vi "main.vi"() -> ()   [LabVIEW 2016]
uses:
  System Status.ctl
  Position Control.ctl
  Position Coordinate.ctl
  Manual Operation Control.ctl
  <vilib>/MakerHub/Xbox-One-Controller/Public/Open First Controller.vi
  <vilib>/MakerHub/Xbox-One-Controller/LMH-Xbox-One-Controller.lvlib
panel:
  in  "Exit Controller":bool
  in  "Use Controller":bool
  out "Numeric 2":dbl
  in  "MotionIni File In":path=path "C:/Program Files (x86)/National Instruments/LabVIEW 2016/user.lib/iselmotion/CNCAPI/CtrlDll/Dummy/MctlDummy.INI"
  in  "MotionLibrary Path":path=path "C:/Program Files (x86)/National Instruments/LabVIEW 2016/user.lib/iselmotion/CNCAPI/CtrlDll/Dummy/mctlDummy.dll"
  in  "Auto Run Control":T1[](array[typedef])
  in  "Auto Run":bool
  in  "Abs Position":T2={"Pos X"=0.0, "Position Name"="Abs Move", "Pos Y"=0.0, "Pos Z"=0.0, "Pos A"=0.0, "OK Button"=FALSE, "Normal Move"=FALSE, "Fast Move"=FALSE} {"Pos A" format="%.2f"; "Pos Z" format="%.2f"; "Pos Y" format="%.2f"; "Pos X" format="%.2f"}
  in  "Rel Position":T2={"Pos X"=0.0, "Position Name"="Rel Move", "Pos Y"=0.0, "Pos Z"=0.0, "Pos A"=0.0, "OK Button"=FALSE, "Normal Move"=FALSE, "Fast Move"=FALSE} {"Pos A" format="%.2f"; "Pos Z" format="%.2f"; "Pos Y" format="%.2f"; "Pos X" format="%.2f"}
  in  "Manual Operation Control":T3={"Pos X"={"Plus"=FALSE, "Minus"=FALSE}, "Pos Y"={"Plus"=FALSE, "Minus"=FALSE}, "Pos Z"={"Plus"=FALSE, "Minus"=FALSE}, "Pos A"={"Plus"=FALSE, "Minus"=FALSE}, "Linear"={"Speed"=1.0, "Step Length"=0.01}, "Rotative"={"Speed"=1.0, "Step Length"=0.01}, "Speed Override (%)"=100.0, "Axis-A Movement"=FALSE} {"Speed Override (%)" min=0.0 max=150.0 step=1.0 scale=0.0..150.0; "Rotative"."Step Length" min=0.01 max=100.0 step=0.01; "Rotative"."Speed" min=0.0 max=500.0 step=1.0 scale=0.0..500.0 scale format="%#.0f"; "Linear"."Step Length" min=0.01 max=500.0 step=0.01; "Linear"."Speed" min=0.0 max=500.0 step=1.0 scale=0.0..500.0 scale format="%#.0f"}
  out "Status":bool
  in  "Test Mode":bool
  in  "Leave HWLS":bool
  in  "Reference":bool
  in  "Reset Motion":bool
  in  "Stop Motion":bool
  in  "Settings":bool
  in  "Exit":bool
  in  "Initialize":bool
  out "System Status":T4 {"Axis A"."Position" format="%.2f"; "Axis Z"."Position" format="%.2f"; "Axis Y"."Position" format="%.2f"; "Rotativ Speed" format="%#_6f"; "Linear Speed" format="%#.2f"; "Axis X"."Position" format="%.2f"}
  out "Error Information":string
  out "Motor hModule":i32
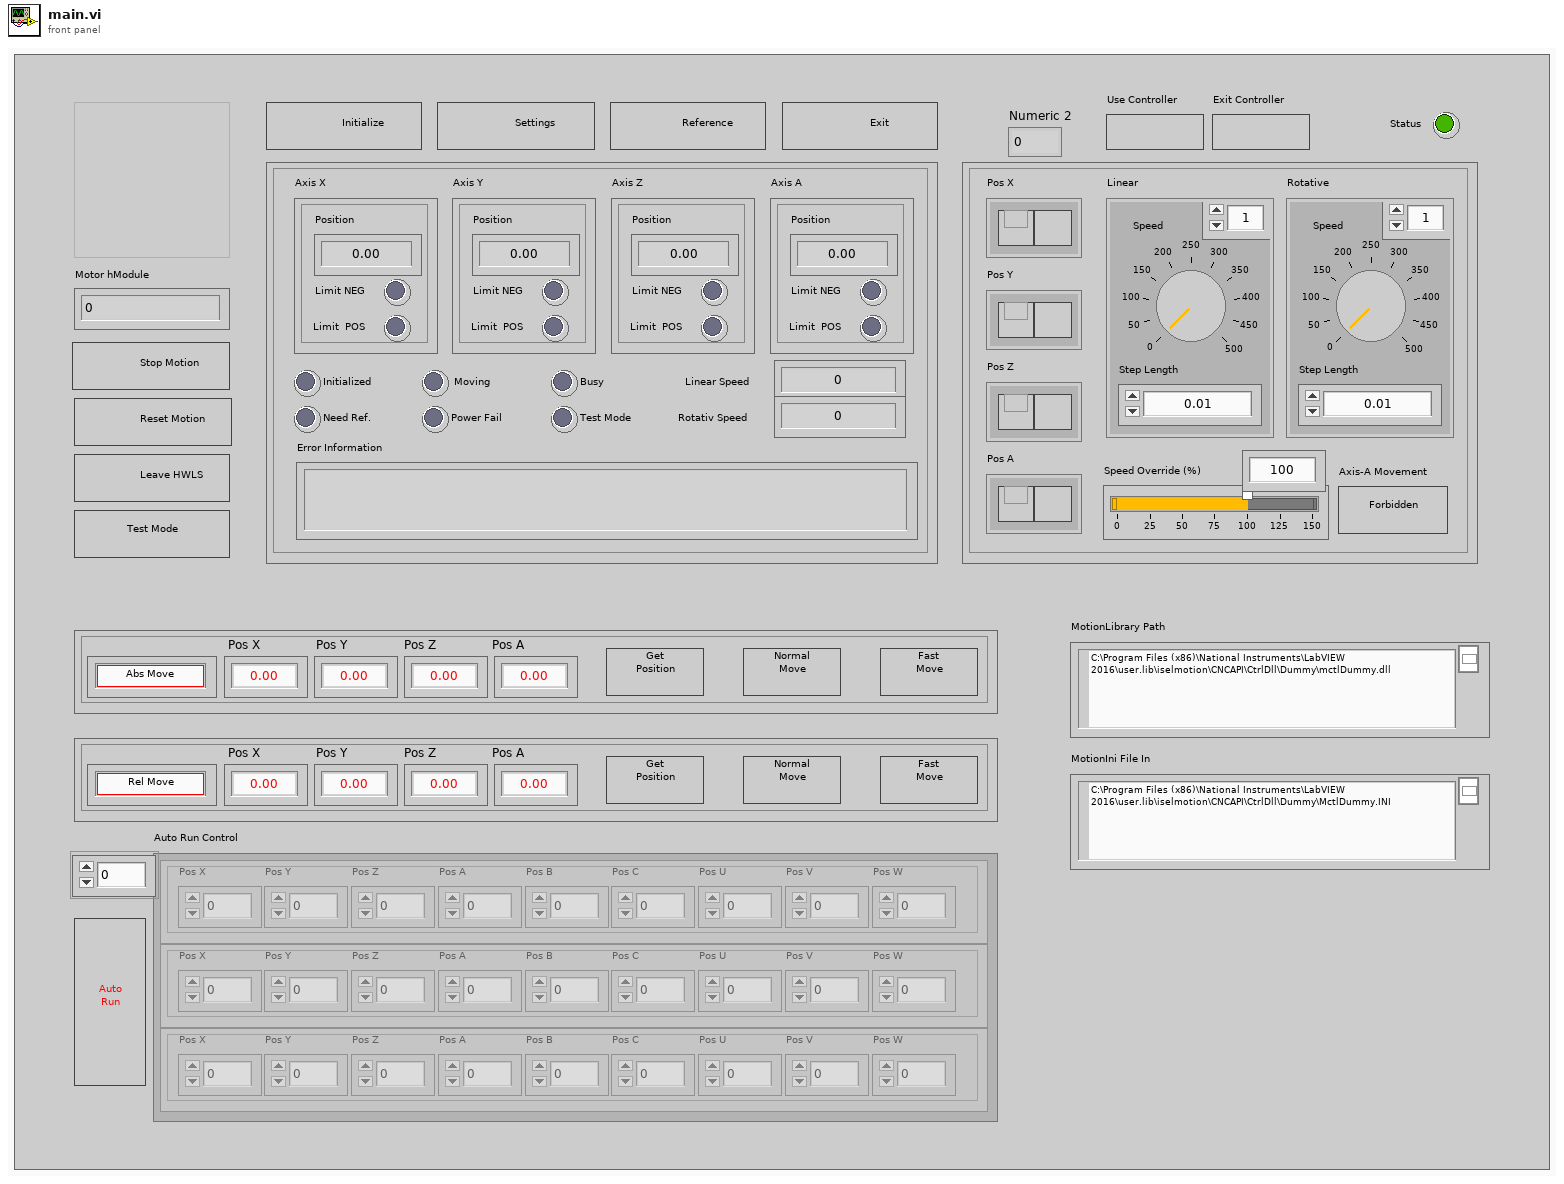
[diagram p1: front panel]
types:
  T1 = typedef "Position Coordinate.ctl" = cluster{"Pos X":dbl, "Pos Y":dbl, "Pos Z":dbl, "Pos A":dbl, "Pos B":dbl, "Pos C":dbl, "Pos U":dbl, "Pos V":dbl, "Pos W":dbl}
  T2 = typedef "Position Control.ctl" = cluster{"Pos X":dbl, "Position Name":string, "Pos Y":dbl, "Pos Z":dbl, "Pos A":dbl, "OK Button":bool, "Normal Move":bool, "Fast Move":bool}
  T3 = typedef "Manual Operation Control.ctl" = cluster{"Pos X":cluster{"Plus":bool, "Minus":bool}, "Pos Y":cluster{"Plus":bool, "Minus":bool}, "Pos Z":cluster{"Plus":bool, "Minus":bool}, "Pos A":cluster{"Plus":bool, "Minus":bool}, "Linear":cluster{"Speed":dbl, "Step Length":dbl}, "Rotative":cluster{"Speed":dbl, "Step Length":dbl}, "Speed Override (%)":dbl, "Axis-A Movement":bool}
  T4 = typedef "System Status.ctl" = cluster{"Axis X":cluster{"Position":dbl, "Limit NEG":bool, "Limit  POS":bool}, "Axis Y":cluster{"Position":dbl, "Limit NEG":bool, "Limit  POS":bool}, "Axis Z":cluster{"Position":dbl, "Limit NEG":bool, "Limit  POS":bool}, "Axis A":cluster{"Position":dbl, "Limit NEG":bool, "Limit  POS":bool}, "Initialized":bool, " Moving":bool, "Busy":bool, "Need Ref.":bool, "Power Fail":bool, "Test Mode":bool, "Linear Speed":dbl, "Rotativ Speed":dbl, "Error Information":string}
  T5 = enum16{"open", "replace", "create", "open or create", "replace or create", "replace or create with confirmation"}
  T6 = enum8{"Enabled", "Disabled", "Disabled and Grayed Out"}
  T7 = cluster{"PosX":i32, "PosY":i32, "PosZ":i32, "PosA":i32, "PosB":i32, "PosC":i32, "PosU":i32, "PosV":i32, "PosW":i32}
  T8 = cluster{"MotionLibrary Path":path, "MotionIni File In":path}
  T9 = typedef "LMH-Xbox-One-Controller.lvlib/Xbox One Controller Ref.ctl" = cluster{"Controller Ref":refnum<k1>, "Event Refnum":refnum<event-registration>, "Worker Ref":refnum<vi>}
  T10 = cluster{"Common":cluster{"INMOTION":bool, "INSTOPMODE":bool, "INTEACHMODE":bool, "INTESTMODE":bool, "CURRENTOFF":bool, "INPATHMOTION":bool, "ISMOVING":bool, "PATHSTARTED":bool, "NEEDREFERENCERUN":bool, "BREAKERROR":bool, "HWLSACTIVE":bool, "SWLSACTIVE":bool, "HWLSDURINGMOTION":bool, "AFTERRUNERROR":bool, "LOADPATHDATAERROR":bool, "KEYSWITCHERROR":bool, "KEYSWDURINGMOTION":bool, "POWER_FAIL":bool, "SC_FAIL":bool, "HARDWARE_FAIL":bool, "COMMUNICATION_FAIL":bool}, "HWLSNeg":cluster{"HWLS_X_NEG":bool, "HWLS_Y_NEG":bool, "HWLS_Z_NEG":bool, "HWLS_A_NEG":bool, "HWLS_B_NEG":bool, "HWLS_C_NEG":bool, "HWLS_U_NEG":bool, "HWLS_V_NEG":bool, "HWLS_W_NEG":bool}, "HWLSPos":cluster{"HWLS_X_POS":bool, "HWLS_Y_POS":bool, "HWLS_Z_POS":bool, "HWLS_A_POS":bool, "HWLS_B_POS":bool, "HWLS_C_POS":bool, "HWLS_U_POS":bool, "HWLS_V_POS":bool, "HWLS_W_POS":bool}, "SWLSNeg":cluster{"SWLS_X_NEG":bool, "SWLS_Y_NEG":bool, "SWLS_Z_NEG":bool, "SWLS_A_NEG":bool, "SWLS_B_NEG":bool, "SWLS_C_NEG":bool, "SWLS_U_NEG":bool, "SWLS_V_NEG":bool, "SWLS_W_NEG":bool}, "SWLSPos":cluster{"SWLS_X_POS":bool, "SWLS_Y_POS":bool, "SWLS_Z_POS":bool, "SWLS_A_POS":bool, "SWLS_B_POS":bool, "SWLS_C_POS":bool, "SWLS_U_POS":bool, "SWLS_V_POS":bool, "SWLS_W_POS":bool}, "Extended":cluster{"ISBUSY":bool, "DISABLED":bool, "ISINITIALIZED":bool, "READY":bool, "DRILLCYCLEACTIVE":bool, "CTRLSPECERROR":bool}, "Additional flags":cluster{"InMotion":bool, "InStopMode":bool, "InTeachMode":bool, "InTestMode":bool, "CurrentOff":bool, "InPathMotion":bool, "IsMoving":bool, "NeedReferenceRun":bool, "BreakError":bool, "HWLSActive":bool, "SWLSActive":bool, "HWLSDuringMotion":bool, "AfterRunError":bool, "PowerFail":bool, "SCFail":bool, "IsBusy":bool, "Initialized":bool, "Disabled":bool, "HardwareFail":bool, "CommunicationFail":bool, "DrillCycleActive":bool, "CtrlSpecError":bool, "PathStarted":bool}}
  T11 = cluster{"PosX":dbl, "PosY":dbl, "PosZ":dbl, "PosA":dbl, "PosB":dbl, "PosC":dbl, "PosU":dbl, "PosV":dbl, "PosW":dbl}
  T12 = cluster{"PosX":dbl, "HWLS_X_NEG":bool, "HWLS_X_POS":bool}
  T13 = cluster{"PosY":dbl, "HWLS_Y_NEG":bool, "HWLS_Y_POS":bool}
  T14 = cluster{"PosZ":dbl, "HWLS_Z_NEG":bool, "HWLS_Z_POS":bool}
  T15 = cluster{dbl, "HWLS_A_NEG":bool, "HWLS_A_POS":bool}
  T16 = cluster{"LiNormVel":i32, "DrNormVel":i32, "LiFastVel":i32, "DrFastVel":i32, "LiTeachVel":i32, "DrTeachVel":i32, "LiActVel":i32, "DrActVel":i32}
  T17 = cluster{"LiNormVel":dbl, "DrNormVel":dbl, "LiFastVel":dbl, "DrFastVel":dbl, "LiTeachVel":dbl, "DrTeachVel":dbl, "LiActVel":dbl, "DrActVel":dbl}
  T18 = typedef "LMH-Xbox-One-Controller.lvlib/All Buttons Visual.ctl" = cluster{"A":T19, "B":T20, "X":T21, "Y":T22, "Left Bumper":T23, "Right Bumper":T24, "View Button":T25, "Menu Button":T26, "Left Stick":T27, "Right Stick":T27}
  T19 = typedef "LMH-Xbox-One-Controller.lvlib/A.ctl" = bool
  T20 = typedef "LMH-Xbox-One-Controller.lvlib/B.ctl" = bool
  T21 = typedef "LMH-Xbox-One-Controller.lvlib/X.ctl" = bool
  T22 = typedef "LMH-Xbox-One-Controller.lvlib/Y.ctl" = bool
  T23 = typedef "LMH-Xbox-One-Controller.lvlib/Left Bumper.ctl" = bool
  T24 = typedef "LMH-Xbox-One-Controller.lvlib/Right Bumper.ctl" = bool
  T25 = typedef "LMH-Xbox-One-Controller.lvlib/View.ctl" = bool
  T26 = typedef "LMH-Xbox-One-Controller.lvlib/Menu.ctl" = bool
  T27 = typedef "LMH-Xbox-One-Controller.lvlib/Thumbstick.ctl" = bool
  T28 = typedef "LMH-Xbox-One-Controller.lvlib/All Axis Data.ctl" = cluster{"Left Stick":cluster{"X Axis":i32, "Y Axis":i32}, "Right Stick":cluster{"X Axis":i32, "Y Axis":i32}, "Triggers":i32, "D-Pad":T29}
  T29 = typedef "LMH-Xbox-One-Controller.lvlib/DPad Enum.ctl" = enum16{"Idle", "Up", "Up / Right", "Right", "Down / Right", "Down", "Down / Left", "Left", "Up / Left"}
  T30 = cluster{"X Axis":i32, "Y Axis":i32, "Y Axis":i32, "Triggers":i32}
  T31 = cluster{"X Axis":bool, "Y Axis":bool, "Y Axis":bool, "Triggers":bool}
  T32 = cluster{"[0]":dbl, "[1]":dbl, "[2]":dbl, "[3]":dbl}
  T33 = cluster{"Ability":cluster{"LINEAR":bool, "CIRCLE":bool, "HELIX":bool, "SPLINE":bool, "BEZIER":bool, "PRECALC":bool, "ONLINE":bool}, "NumAxis":u32, "AxisConfig":cluster{"AxisConfig 0":cluster{"Type":cluster{"LINEAR":bool, "ROT":bool}, "In Use":bool, "ID":u32, "RangeMin":u32, "RangeMax":u32}, "AxisConfig 1":cluster{"Type":cluster{"LINEAR":bool, "ROT":bool}, "In Use":bool, "ID":u32, "RangeMin":u32, "RangeMax":u32}, "AxisConfig 2":cluster{"Type":cluster{"LINEAR":bool, "ROT":bool}, "In Use":bool, "ID":u32, "RangeMin":u32, "RangeMax":u32}, "AxisConfig 3":cluster{"Type":cluster{"LINEAR":bool, "ROT":bool}, "In Use":bool, "ID":u32, "RangeMin":u32, "RangeMax":u32}, "AxisConfig 4":cluster{"Type":cluster{"LINEAR":bool, "ROT":bool}, "In Use":bool, "ID":u32, "RangeMin":u32, "RangeMax":u32}, "AxisConfig 5":cluster{"Type":cluster{"LINEAR":bool, "ROT":bool}, "In Use":bool, "ID":u32, "RangeMin":u32, "RangeMax":u32}, "AxisConfig 6":cluster{"Type":cluster{"LINEAR":bool, "ROT":bool}, "In Use":bool, "ID":u32, "RangeMin":u32, "RangeMax":u32}, "AxisConfig 7":cluster{"Type":cluster{"LINEAR":bool, "ROT":bool}, "In Use":bool, "ID":u32, "RangeMin":u32, "RangeMax":u32}, "AxisConfig 8":cluster{"Type":cluster{"LINEAR":bool, "ROT":bool}, "In Use":bool, "ID":u32, "RangeMin":u32, "RangeMax":u32}}}
  T34 = cluster{"In Use":bool, "In Use":bool, "In Use":bool, "In Use":bool, "In Use":bool, "In Use":bool, "In Use":bool, "In Use":bool, "In Use":bool}
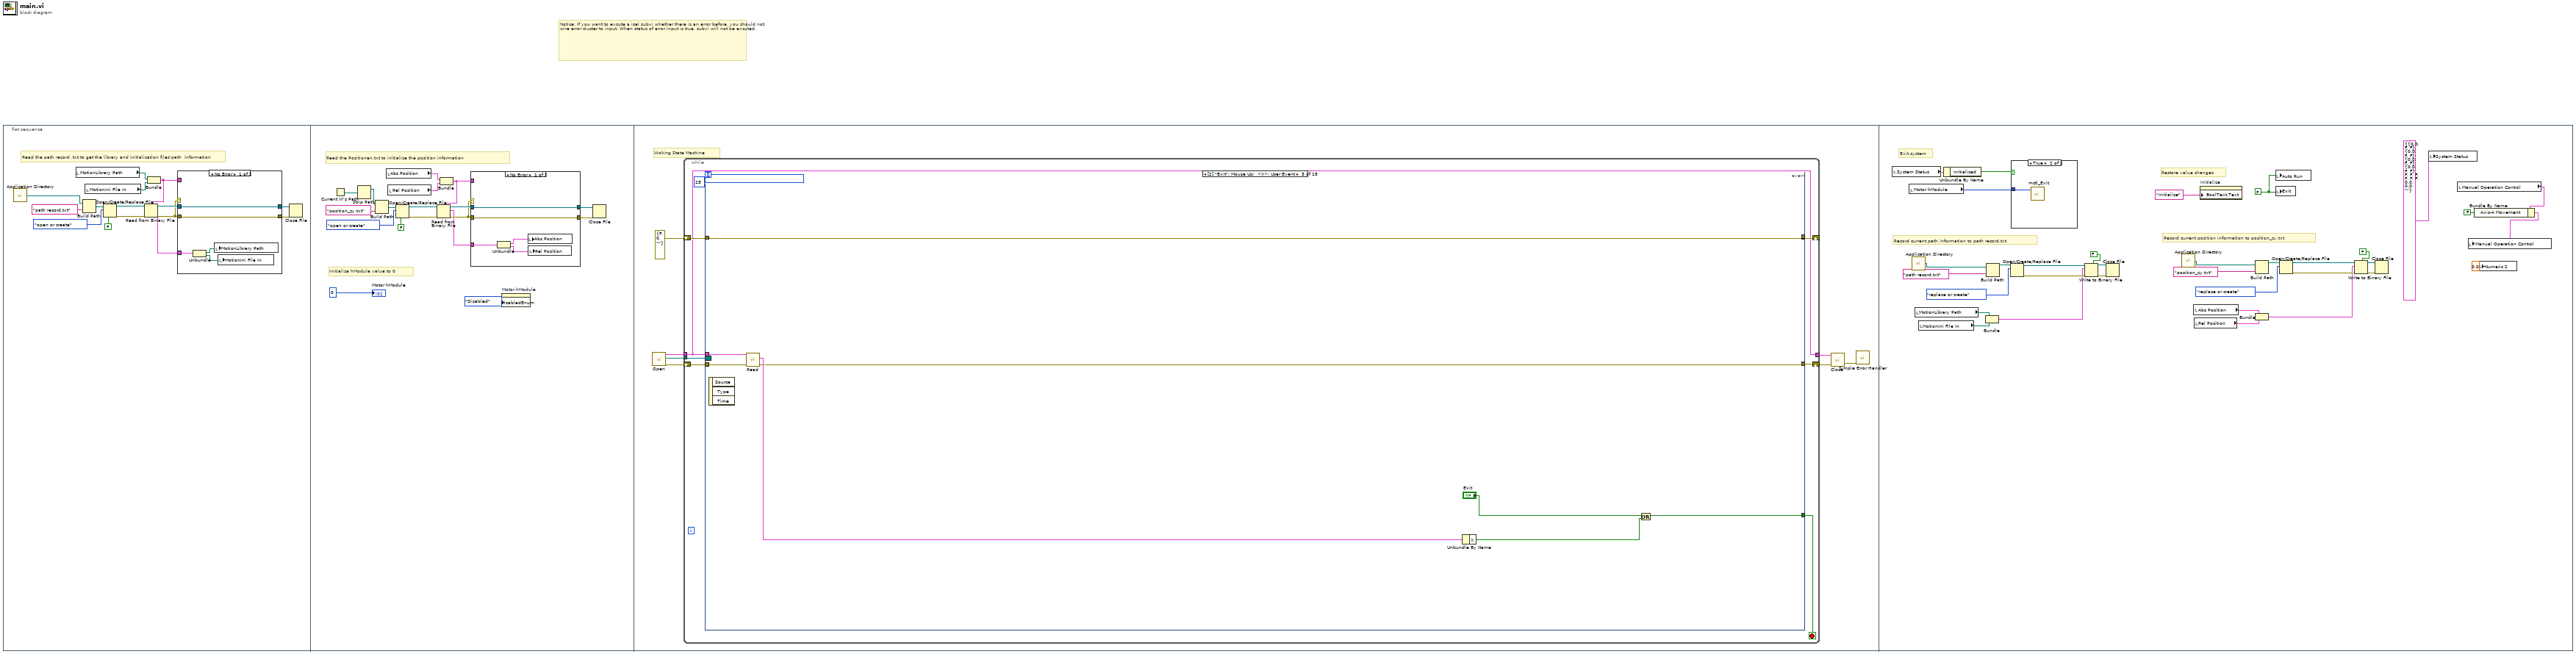
[diagram p0: block diagram]
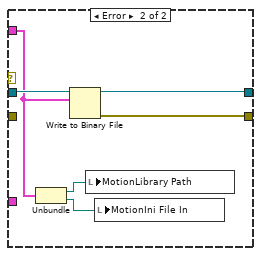
[diagram p2: hidden frame]
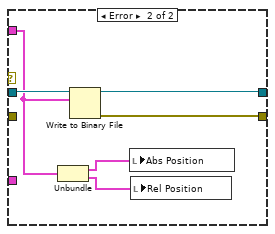
[diagram p3: hidden frame]
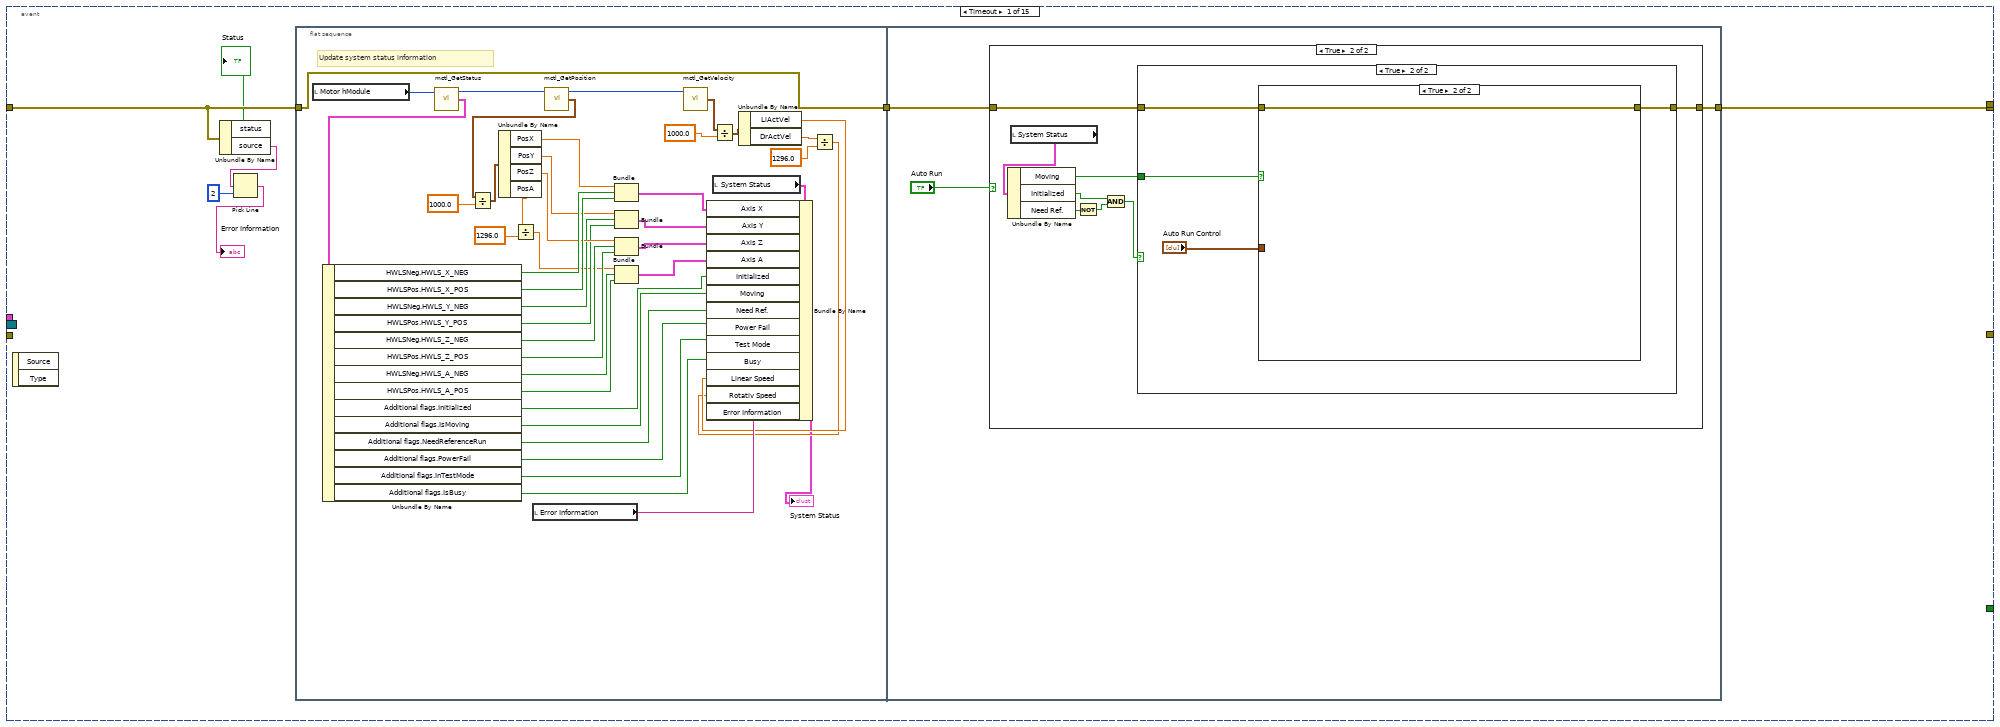
[diagram p4: hidden frame]
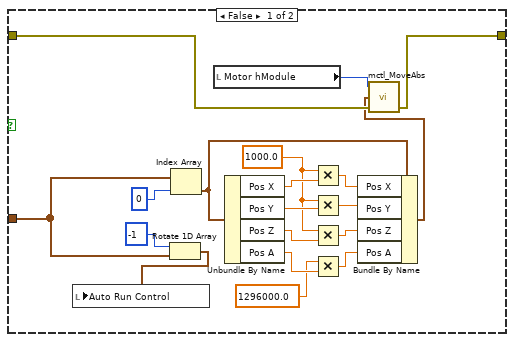
[diagram p7: hidden frame]
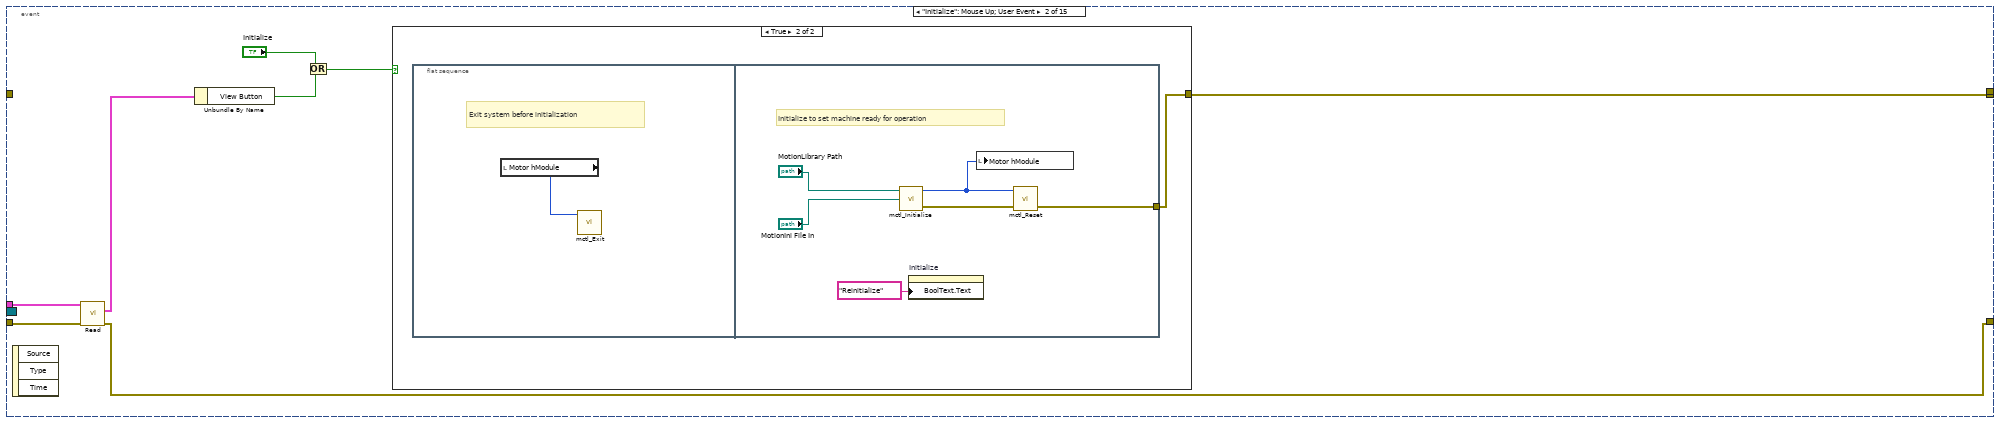
[diagram p8: hidden frame]
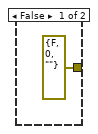
[diagram p9: hidden frame]
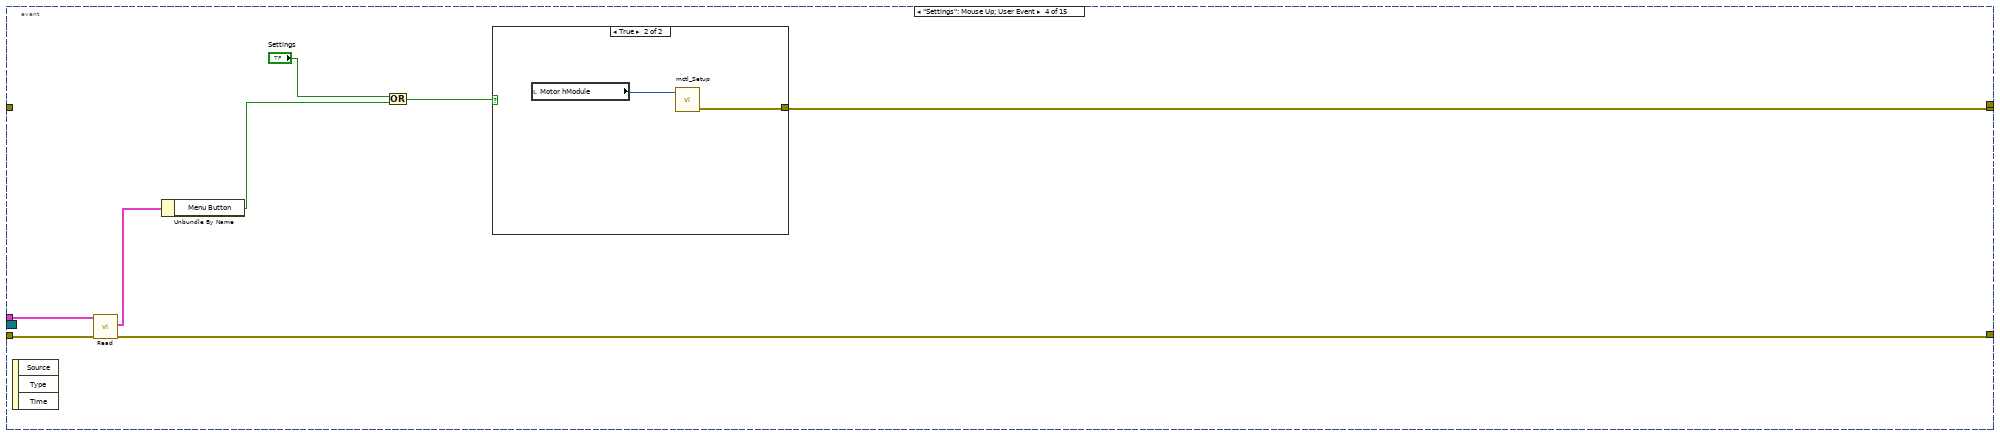
[diagram p10: hidden frame]
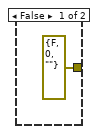
[diagram p11: hidden frame]
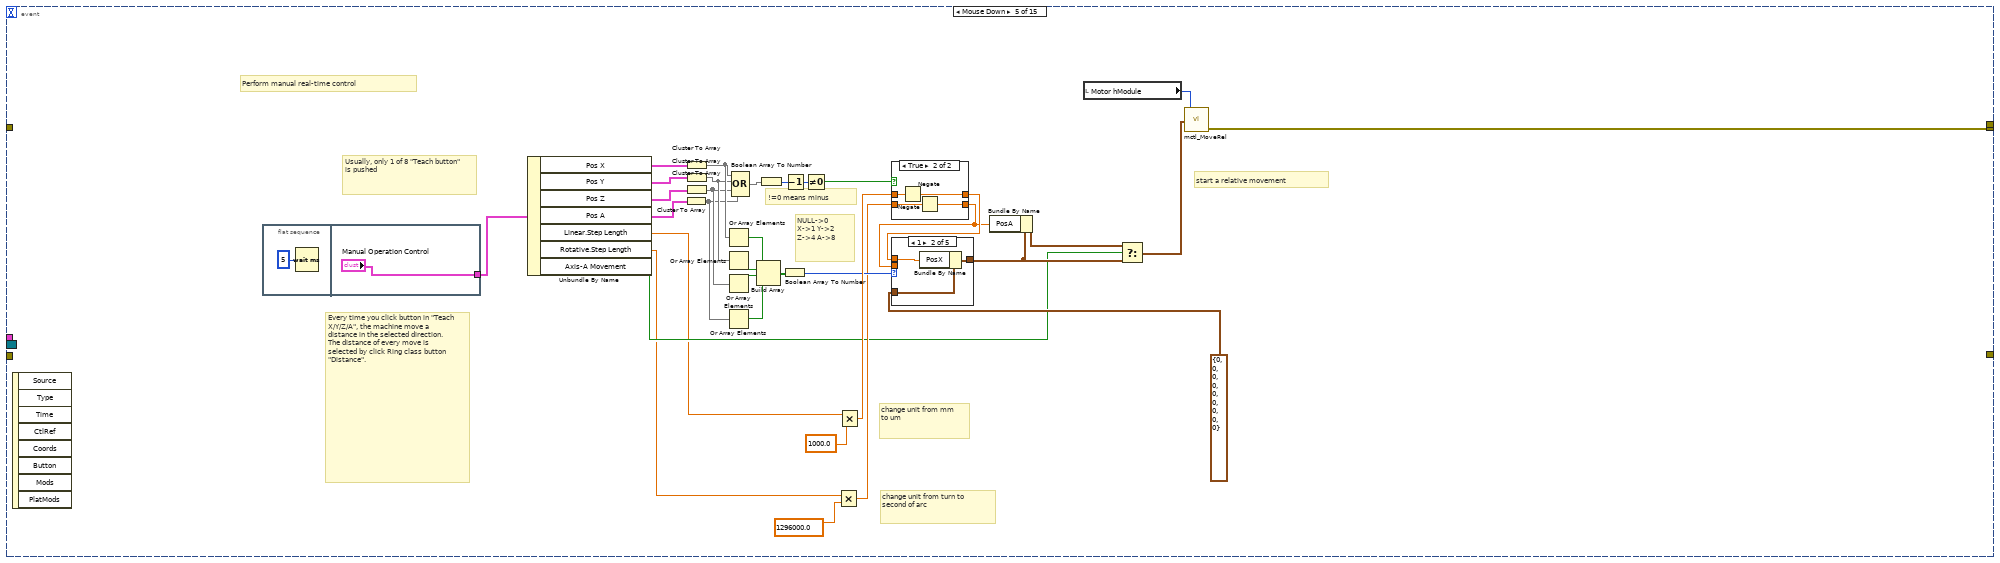
[diagram p12: hidden frame]
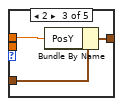
[diagram p14: hidden frame]
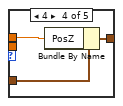
[diagram p15: hidden frame]
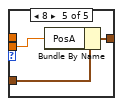
[diagram p16: hidden frame]
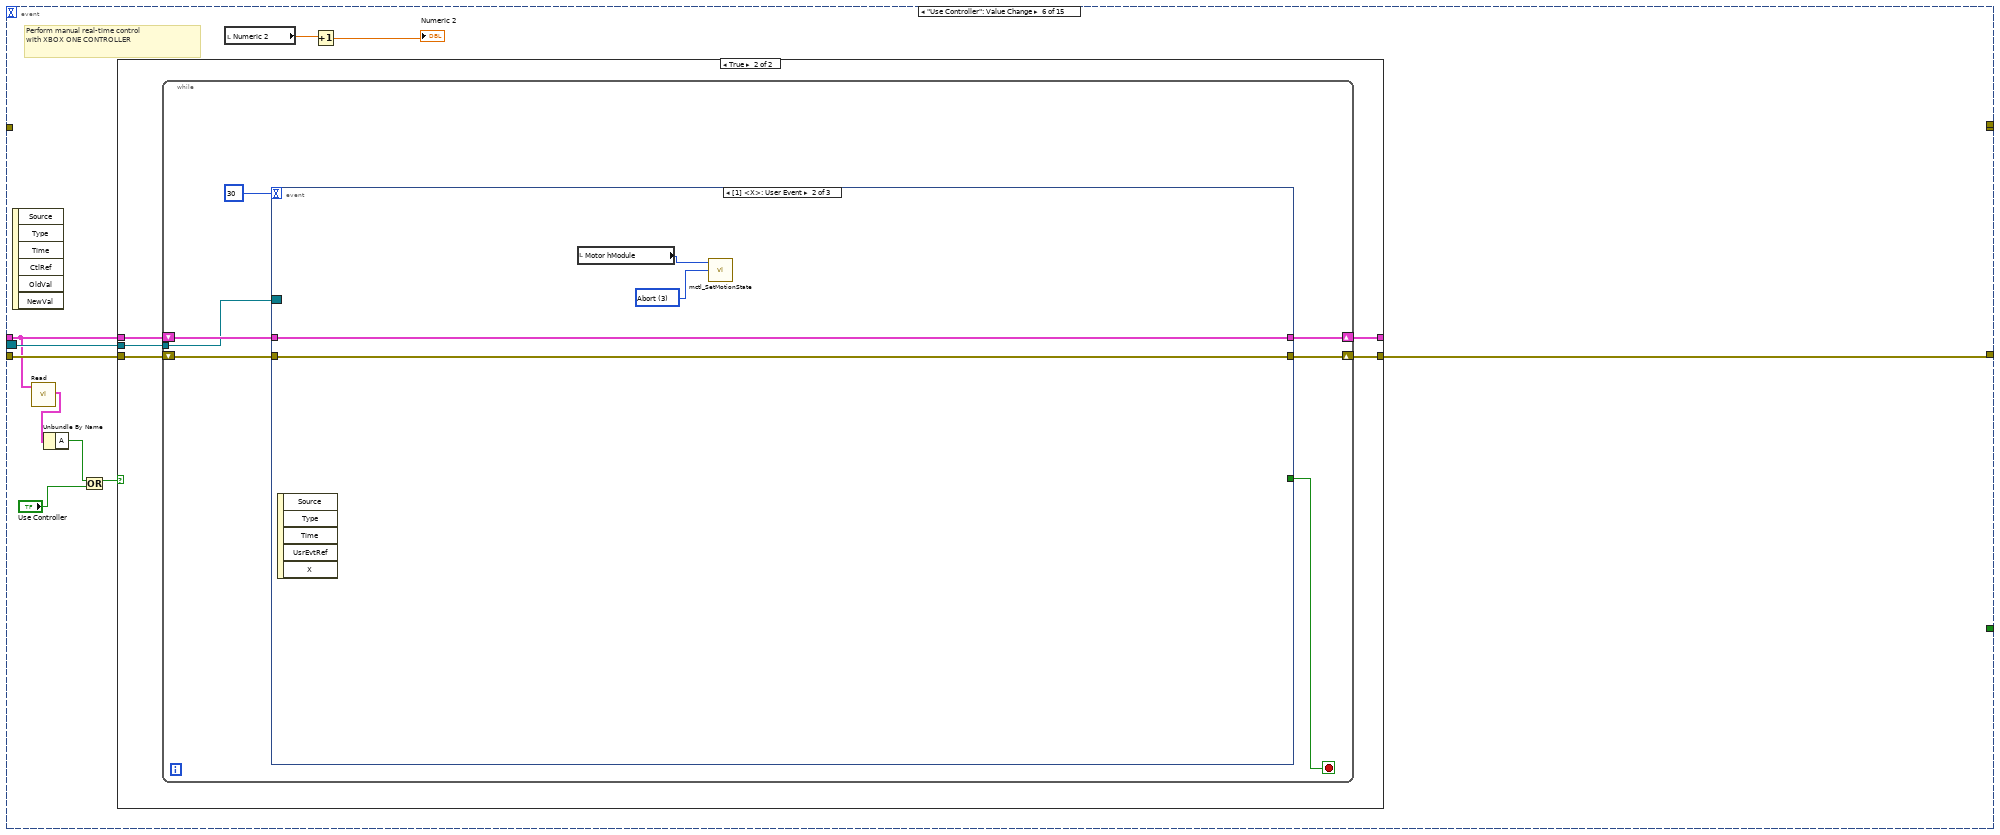
[diagram p18: hidden frame]
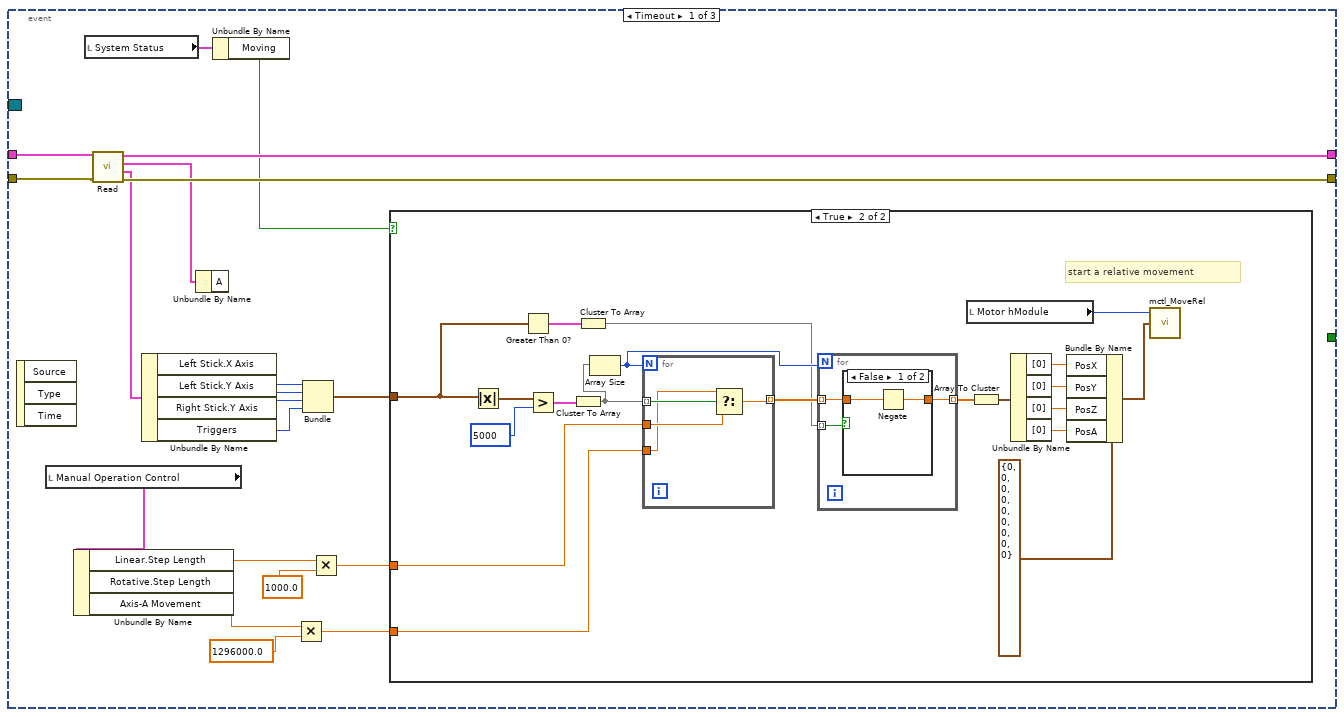
[diagram p20: hidden frame]
diagram:
  # "Notice: If you want to excute a isel subvi whether there is an error before, you should not wire error cluster to input. When status of error input is true, subvi will not be excuted."
  n1 = flat-sequence {
    frame #0 {
      # "Read the path record .txt to get the library and initialization files'path  information"
      n2 = call <vilib>:"Application Directory.vi"() -> ("Application Directory"=w2:path)
      n3 = local read "MotionLibrary Path"() -> (w10:path)
      n4 = Build Path(base path=w2, name or relative path="path record.txt") -> (appended path=w13:path)
      n5 = local read "MotionIni File In"() -> (w11:path)
      n6 = Open/Create/Replace File(file path (use dialog)=w13, operation (0:open)=T5."open or create", disable buffering (F)=FALSE ("advisory dialog? (display:T)")) -> (refnum out=w15:refnum<file>, error out=w12:errorcluster)  [unwired: 3 in, 1 out]
      n7 = Bundle("MotionLibrary Path"=w10, "MotionIni File In"=w11) -> (w3:T8)  [unwired: 1 in]
      n8 = Read from Binary File(5:w3, 8:w12, 11:w15) -> (0:w4:errorcluster, 2:w1:T8, 3:w7:refnum<file>)  [unwired: 3 in, 1 out]
      n9 = case shown="No Error" w4 {
        tunnel: w7 -> [w20 w26]
        tunnel: [w20 w24] -> w6
        tunnel: [w19 w25] -> w5
        tunnel: w4 -> [w19 _]
        tunnel: w3 -> [_ w23]
        tunnel: w1 -> [w18 _]
        frame No Error {
          n10 = Unbundle(w18) -> ("MotionLibrary Path"=w17:path, "MotionIni File In"=w16:path)
          n11 = local write "MotionLibrary Path"(w17) -> ()
          n12 = local write "MotionIni File In"(w16) -> ()
        }
        frame Error {
          n13 = Unbundle(w23) -> ("MotionLibrary Path"=w22:path, "MotionIni File In"=w21:path)
          n14 = Write to Binary File(file (use dialog)=w26, data=w23) -> (refnum out=w24:refnum<file>, error out=w25:errorcluster)  [unwired: 4 in, 1 out]
          n15 = local write "MotionLibrary Path"(w22) -> ()
          n16 = local write "MotionIni File In"(w21) -> ()
        }
      }
      n17 = Close File(refnum=w6, error in=w5) -> ()  [unwired: 2 out]
    }
    frame #1 {
      # "Initialize hModule value to 0"
      # "Read the Positionen.txt to initialize the position information"
      n18 = Current VI's Path() -> (path=w30:path)
      n19 = Strip Path(path=w30) -> (stripped path=w43:path)  [unwired: 1 out]
      n20 = Build Path(base path=w43, name or relative path="position_zy.txt") -> (appended path=w41:path)
      n21 = local read "Abs Position"() -> (w38:T2)
      n22 = local read "Rel Position"() -> (w39:T2)
      n23 = Open/Create/Replace File(file path (use dialog)=w41, operation (0:open)=T5."open or create", disable buffering (F)=FALSE ("advisory dialog? (display:T)")) -> (refnum out=w44:refnum<file>, error out=w40:errorcluster)  [unwired: 3 in, 1 out]
      n24 = Bundle("Abs Position"=w38, "Rel Position"=w39) -> (w31:cluster{"Abs Position":T2, "Rel Position":T2})  [unwired: 1 in]
      n25 = Read from Binary File(5:w31, 8:w40, 11:w44) -> (0:w32:errorcluster, 2:w28:cluster{"Abs Position":T2, "Rel Position":T2}, 3:w35:refnum<file>)  [unwired: 3 in, 1 out]
      n26 = case shown="No Error" w32 {
        tunnel: w35 -> [w49 w55]
        tunnel: [w49 w53] -> w34
        tunnel: [w48 w54] -> w33
        tunnel: w32 -> [w48 _]
        tunnel: w31 -> [_ w52]
        tunnel: w28 -> [w47 _]
        frame No Error {
          n27 = Unbundle(w47) -> ("Abs Position"=w46:T2, "Rel Position"=w45:T2)
          n28 = local write "Abs Position"(w46) -> ()
          n29 = local write "Rel Position"(w45) -> ()
        }
        frame Error {
          n30 = Unbundle(w52) -> ("Abs Position"=w51:T2, "Rel Position"=w50:T2)
          n31 = Write to Binary File(file (use dialog)=w55, data=w52) -> (refnum out=w53:refnum<file>, error out=w54:errorcluster)  [unwired: 4 in, 1 out]
          n32 = local write "Abs Position"(w51) -> ()
          n33 = local write "Rel Position"(w50) -> ()
        }
      }
      n34 = property on="Motor hModule" class="DigNum (strict)"("DisabledEnum"=T6."Disabled" ("Disabled")) -> ()  [unwired: 2 in, 2 out]
      n35 = Close File(refnum=w34, error in=w33) -> ()  [unwired: 2 out]
      "Motor hModule" <- 0
    }
    frame #2 {
      # "Woking State Machine"
      n36 = call-poly <vilib>:"Open.vi"() -> ("Error Out"=w59:errorcluster, "Event Refnum"=w61:refnum<event-registration>, "Xbox One Controller"=w60:T9)  [unwired: 9 in]
      n37 = while {
        shift-right: [w68] -> _
        shift-left: errorcluster {"status"=FALSE, "code"=0, "source"=""} ("error constant") -> [w69]
        tunnel: w61 -> [w66]
        shift-right: [w64] -> w58
        shift-left: w59 -> [w65]
        tunnel: w60 -> [w63]
        tunnel: [w63] -> w57
        stop <- w67 stop-if-true
        n38 = event shown="[2] \"Exit\": Mouse Up;  <X>: User Event" {
          selector: w66 -> [_ _ _ _ _ w257 _ _ _ _ _ _ _ _ _]
          dyn-events: _ -> [_ _ _ _ _ _ _ _ _ _ _ _ _ _ _]
          timeout: 25 -> [_ _ _ _ _ _ _ _ _ _ _ _ _ _ _]
          tunnel: w69 -> [w77 _ w180 _ _ _ w335 _ _ _ _ _ w411 w461 _]
          tunnel: [w72 w164 w180 w189 w195 _ w334 w336 w341 w349 w394 w403 _ w460 w511] -> w68
          tunnel: [_ _ w175 _ _ _ _ _ _ _ _ _ _ _ _] -> w67
          tunnel: [_ _ _ _ _ _ _ _ _ _ _ _ w410 _ _] -> _
          tunnel: w63 -> [_ w163 w178 w188 _ w255 _ _ _ w347 _ _ _ _ _]
          tunnel: w65 -> [_ w162 w177 w187 _ w256 _ _ _ w346 _ _ _ _ _]
          tunnel: [_ w157 w176 w182 _ w252 _ _ _ _ _ _ _ _ _] -> w64
          event Timeout {
            n39 = event-data() -> ()  [unwired: 1 in, 2 out]
            n40 = Unbundle By Name(w77) -> ("status"=→"Status":bool, "source"=w75:string)
            n41 = Pick Line(multi-line string=w75, line index=2) -> (output string=→"Error Information":string)  [unwired: 1 in]
            n42 = flat-sequence {
              tunnel: w77 -> [w79]
              tunnel: [w79] -> w73
              tunnel: w73 -> [w121]
              tunnel: [w120] -> w72
              frame #0 {
                # "Update system status information"
                n43 = local read "Motor hModule"() -> (w119:i32)
                n44 = call <userlib>:"mctl_GetStatus.vi"("hModule In"=w119) -> ("Status"=w118:T10, "hModule Out"=w117:u32)  [unwired: 2 in, 1 out]
                n45 = Unbundle By Name(w118) -> ("HWLSNeg.HWLS_X_NEG"=w111:bool, "HWLSPos.HWLS_X_POS"=w110:bool, "HWLSNeg.HWLS_Y_NEG"=w107:bool, "HWLSPos.HWLS_Y_POS"=w106:bool, "HWLSNeg.HWLS_Z_NEG"=w105:bool, "HWLSPos.HWLS_Z_POS"=w104:bool, "HWLSNeg.HWLS_A_NEG"=w103:bool, "HWLSPos.HWLS_A_POS"=w102:bool, "Additional flags.Initialized"=w97:bool, "Additional flags.IsMoving"=w96:bool, "Additional flags.NeedReferenceRun"=w95:bool, "Additional flags.PowerFail"=w92:bool, "Additional flags.InTestMode"=w93:bool, "Additional flags.IsBusy"=w94:bool)
                n46 = local read "Error Information"() -> (w91:string)
                n47 = call <userlib>:"mctl_GetPosition.vi"("hModule In"=w117) -> ("AxisPos"=w115:T7, "hModule Out"=w116:u32)  [unwired: 2 in, 1 out]
                n48 = Divide(x=w115, y=1000.0) -> (x/y=w113:T11)
                n49 = Unbundle By Name(w113) -> ("PosX"=w112:dbl, "PosY"=w109:dbl, "PosZ"=w108:dbl, "PosA"=w89:dbl)
                n50 = Divide(x=w89, y=1296.0) -> (x/y=w87:dbl)
                n51 = Bundle("PosX"=w112, "HWLS_X_NEG"=w111, "HWLS_X_POS"=w110) -> (w101:T12)  [unwired: 1 in]
                n52 = Bundle("PosY"=w109, "HWLS_Y_NEG"=w107, "HWLS_Y_POS"=w106) -> (w100:T13)  [unwired: 1 in]
                n53 = Bundle("PosZ"=w108, "HWLS_Z_NEG"=w105, "HWLS_Z_POS"=w104) -> (w99:T14)  [unwired: 1 in]
                n54 = Bundle(w87, "HWLS_A_NEG"=w103, "HWLS_A_POS"=w102) -> (w98:T15)  [unwired: 1 in]
                n55 = call <userlib>:"mctl_GetVelocity.vi"("hModule In"=w116) -> ("Velocity"=w84:T16)  [unwired: 2 in, 2 out]
                n56 = Divide(x=w84, y=1000.0) -> (x/y=w85:T17)
                n57 = local read "System Status"() -> (w90:T4)
                n58 = Unbundle By Name(w85) -> ("LiActVel"=w86:dbl, "DrActVel"=w82:dbl)
                n59 = Divide(x=w82, y=1296.0) -> (x/y=w80:dbl)
                n60 = Bundle By Name(cluster=w90, "Axis X"=w101, "Axis Y"=w100, "Axis Z"=w99, "Axis A"=w98, "Initialized"=w97, "Moving"=w96, "Need Ref."=w95, "Power Fail"=w92, "Test Mode"=w93, "Busy"=w94, "Linear Speed"=w86, "Rotativ Speed"=w80, "Error Information"=w91) -> (→"System Status":T4)
              }
              frame #1 {
                n61 = case shown="True" "Auto Run" {
                  tunnel: w121 -> [w123 w130]
                  tunnel: [w123 w129] -> w120
                  frame False {
                  }
                  frame True {
                    n62 = local read "System Status"() -> (w131:T4)
                    n63 = Unbundle By Name(w131) -> ("Moving"=w128:bool, "Initialized"=w126:bool, "Need Ref."=w127:bool)
                    n64 = Not(x=w127) -> (.not. x?=w124:bool)
                    n65 = And(x=w126, y=w124) -> (x .and. y?=w125:bool)
                    n66 = case shown="True" w125 {
                      tunnel: w130 -> [w132 w136]
                      tunnel: [w132 w133] -> w129
                      tunnel: w128 -> [_ w134]
                      frame False {
                      }
                      frame True {
                        n67 = case shown="True" w134 {
                          tunnel: w136 -> [w153 w156]
                          tunnel: [w150 w156] -> w133
                          tunnel: "Auto Run Control" -> [w151 _]
                          frame False {
                            w144 = 1000.0
                            n68 = Rotate 1D Array(1:w151, 2:-1 ("n")) -> (0:w149:T1[])
                            n69 = local write "Auto Run Control"(w149) -> ()
                            n70 = Index Array(array=w151, index=0) -> (element=w142:T1)
                            n71 = local read "Motor hModule"() -> (w152:i32)
                            n72 = Unbundle By Name(w142) -> ("Pos X"=w148:dbl, "Pos Y"=w147:dbl, "Pos Z"=w146:dbl, "Pos A"=w145:dbl)
                            n73 = Multiply(x=w144, y=w148) -> (x*y=w141:dbl)
                            n74 = Multiply(x=w144, y=w147) -> (x*y=w140:dbl)
                            n75 = Multiply(x=w144, y=w146) -> (x*y=w139:dbl)
                            n76 = Multiply(x=1296000.0, y=w145) -> (x*y=w138:dbl)
                            n77 = Bundle By Name(cluster=w142, "Pos X"=w141, "Pos Y"=w140, "Pos Z"=w139, "Pos A"=w138) -> (w137:T1)
                            n78 = call <userlib>:"mctl_MoveAbs.vi"("error in"=w153, "Abs"=w137, "hModule In"=w152) -> ("error out"=w150:errorcluster)  [unwired: 1 in, 1 out]
                          }
                          frame True {
                          }
                        }
                      }
                    }
                  }
                }
              }
            }
          }
          event "Initialize": Mouse Up; User Event {
            n79 = event-data() -> ()  [unwired: 1 in, 3 out]
            n80 = call <vilib>:"Read.vi"("Error In"=w162, "Xbox One Controller Ref"=w163) -> ("Error Out"=w157:errorcluster, "Buttons"=w161:T18)  [unwired: 6 in, 2 out]
            n81 = Unbundle By Name(w161) -> ("View Button"=w159:T25)
            n82 = Or(x="Initialize", y=w159) -> (x .or. y?=w158:T25)
            n83 = case shown="True" w158 {
              tunnel: [errorcluster {"status"=FALSE, "code"=0, "source"=""} ("error out") w166] -> w164
              frame False {
              }
              frame True {
                n84 = flat-sequence {
                  tunnel: [w172] -> w166
                  frame #0 {
                    # "Exit system before initialization"
                    n85 = local read "Motor hModule"() -> (w167:i32)
                    n86 = call <userlib>:"mctl_Exit.vi"("hModule In"=w167) -> ()  [unwired: 3 in, 2 out]
                  }
                  frame #1 {
                    # "Initialize to set machine ready for operation"
                    n87 = call <userlib>:"mctl_Initialize.vi"("Ini File In"="MotionIni File In", "Library In"="MotionLibrary Path") -> ("error out"=w173:errorcluster, "hModule Out"=w169:u32)  [unwired: 1 in, 1 out]
                    n88 = property on="Initialize" class="Bool (strict)"("BoolText.Text"="Reinitialize" ("Boolean Text.Text")) -> ()  [unwired: 2 in, 2 out]
                    n89 = local write "Motor hModule"(w169) -> ()
                    n90 = call <userlib>:"mctl_Reset.vi"("error in"=w173, "hModule In"=w169) -> ("error out"=w172:errorcluster)  [unwired: 2 in, 1 out]
                  }
                }
              }
            }
          }
          event "Exit": Mouse Up; User Event {
            n91 = event-data() -> ()  [unwired: 1 in, 3 out]
            n92 = call <vilib>:"Read.vi"("Error In"=w177, "Xbox One Controller Ref"=w178) -> ("Error Out"=w176:errorcluster, "Buttons"=w179:T18)  [unwired: 6 in, 2 out]
            n93 = Unbundle By Name(w179) -> ("X"=w174:T21)
            n94 = Or(x="Exit", y=w174) -> (x .or. y?=w175:T21)
          }
          event "Settings": Mouse Up; User Event {
            n95 = event-data() -> ()  [unwired: 1 in, 3 out]
            n96 = call <vilib>:"Read.vi"("Error In"=w187, "Xbox One Controller Ref"=w188) -> ("Error Out"=w182:errorcluster, "Buttons"=w186:T18)  [unwired: 6 in, 2 out]
            n97 = Unbundle By Name(w186) -> ("Menu Button"=w184:T26)
            n98 = Or(x="Settings", y=w184) -> (x .or. y?=w183:T26)
            n99 = case shown="True" w183 {
              tunnel: [errorcluster {"status"=FALSE, "code"=0, "source"=""} ("error out") w191] -> w189
              frame False {
              }
              frame True {
                n100 = local read "Motor hModule"() -> (w192:i32)
                n101 = call <userlib>:"mctl_Setup.vi"("hModule In"=w192) -> ("error out"=w191:errorcluster)  [unwired: 3 in, 1 out]
              }
            }
          }
          event Mouse Down {
            # "Usually, only 1 of 8 \"Teach button\" is pushed"
            # "!=0 means minus"
            # "change unit from turn to second of arc"
            # "change unit from mm to um"
            # "start a relative movement"
            # "Every time you click button in \"Teach X/Y/Z/A\", the machine move a distance in the selected direction. The distance of every move is selected by click Ring class button \"Distance\"."
            # "NULL->0\nX->1 Y->2\nZ->4 A->8"
            # "Perform manual real-time control"
            n102 = event-data() -> ()  [unwired: 1 in, 8 out]
            n103 = flat-sequence {
              tunnel: ["Manual Operation Control"] -> w198
              frame #0 {
                n104 = Wait (ms)(milliseconds to wait=u32 5) -> ()  [unwired: 1 out]
              }
              frame #1 {
              }
            }
            n105 = Unbundle By Name(w198) -> ("Pos X"=w226:cluster{"Plus":bool, "Minus":bool}, "Pos Y"=w225:cluster{"Plus":bool, "Minus":bool}, "Pos Z"=w224:cluster{"Plus":bool, "Minus":bool}, "Pos A"=w223:cluster{"Plus":bool, "Minus":bool}, "Linear.Step Length"=w194:dbl, "Rotative.Step Length"=w193:dbl, "Axis-A Movement"=w199:bool)
            n106 = Cluster To Array(cluster=w223) -> (array=w214:bool[])
            n107 = Cluster To Array(cluster=w226) -> (array=w217:bool[])
            n108 = Cluster To Array(cluster=w225) -> (array=w216:bool[])
            n109 = Cluster To Array(cluster=w224) -> (array=w215:bool[])
            n110 = Or Array Elements(Boolean array=w217) -> (logical OR=w222:bool)
            n111 = Or Array Elements(Boolean array=w216) -> (logical OR=w221:bool)
            n112 = Or Array Elements(Boolean array=w215) -> (logical OR=w220:bool)
            n113 = Or Array Elements(Boolean array=w214) -> (logical OR=w219:bool)
            n114 = Compound Arithmetic op=OR(w217, w216, w215, w214) -> (w211:bool[])
            n115 = Build Array(w222, w221, w220, w219) -> (w218:bool[])
            n116 = Boolean Array To Number(Boolean array=w211) -> (number=w213:u32)
            n117 = Boolean Array To Number(Boolean array=w218) -> (number=w208:u32)
            n118 = Decrement(x=w213) -> (x-1=w212:u32)
            n119 = Not Equal To 0?(x=w212) -> (x != 0?=w197:bool)
            n120 = Multiply(x=w193, y=1296000.0) -> (x*y=w204:dbl)
            n121 = Multiply(x=w194, y=1000.0) -> (x*y=w209:dbl)
            n122 = case shown="True" w197 {
              tunnel: w209 -> [w243 w247]
              tunnel: [w243 w246] -> w206
              tunnel: w204 -> [w242 w245]
              tunnel: [w242 w244] -> w202
              frame False {
              }
              frame True {
                n123 = Negate(x=w247) -> (-x=w246:dbl)
                n124 = Negate(x=w245) -> (-x=w244:dbl)
              }
            }
            n125 = case shown="1" w208 {
              tunnel: T7 {"PosX"=0, "PosY"=0, "PosZ"=0, "PosA"=0, "PosB"=0, "PosC"=0, "PosU"=0, "PosV"=0, "PosW"=0} ("RelPOS") -> [w229 w231 w234 w237 w240]
              tunnel: [w229 w232 w235 w238 w241] -> w203
              tunnel: w206 -> [_ w230 w233 w236 _]
              tunnel: w202 -> [_ _ _ _ w239]
              frame 0, Default {
              }
              frame 1 {
                n126 = Bundle By Name(cluster=w231, "PosX"=w230) -> (w232:T7)
              }
              frame 2 {
                n127 = Bundle By Name(cluster=w234, "PosY"=w233) -> (w235:T7)
              }
              frame 4 {
                n128 = Bundle By Name(cluster=w237, "PosZ"=w236) -> (w238:T7)
              }
              frame 8 {
                n129 = Bundle By Name(cluster=w240, "PosA"=w239) -> (w241:T7)
              }
            }
            n130 = Bundle By Name(cluster=w203, "PosA"=w202) -> (w201:T7)
            n131 = local read "Motor hModule"() -> (w196:i32)
            n132 = Select(t=w201, s=w199, f=w203) -> (s? t:f=w200:T7)
            n133 = call <userlib>:"mctl_MoveRel.vi"("RelPOS"=w200, "hModule In"=w196) -> ("error out"=w195:errorcluster)  [unwired: 2 in, 1 out]
          }
          event "Use Controller": Value Change {
            # "Perform manual real-time control\nwith XBOX ONE CONTROLLER"
            n134 = event-data() -> ()  [unwired: 1 in, 6 out]
            n135 = call <vilib>:"Read.vi"("Xbox One Controller Ref"=w255) -> ("Buttons"=w254:T18)  [unwired: 7 in, 3 out]
            n136 = Unbundle By Name(w254) -> ("A"=w253:T19)
            n137 = Or(x=w253, y="Use Controller") -> (x .or. y?=w251:T19)
            n138 = case shown="True" w251 {
              tunnel: w257 -> [_ w264]
              tunnel: w255 -> [w259 w263]
              tunnel: w256 -> [w258 w262]
              tunnel: [w259 w261] -> _
              tunnel: [w258 w260] -> w252
              frame False {
              }
              frame True {
                n139 = while {
                  tunnel: w264 -> [w270]
                  shift-right: [w266] -> w261
                  shift-left: w263 -> [w271]
                  shift-right: [w265] -> w260
                  shift-left: w262 -> [w269]
                  stop <- w267 stop-if-true
                  n140 = event shown="[1] <X>: User Event" {
                    selector: w270 -> [_ _ _]
                    dyn-events: _ -> [_ _ _]
                    timeout: 30 -> [_ _ _]
                    tunnel: w271 -> [w291 w325 w330]
                    tunnel: w269 -> [w290 w324 w331]
                    tunnel: [_ _ w327] -> w267
                    tunnel: [w288 w325 w330] -> w266
                    tunnel: [w289 w324 w331] -> w265
                    event Timeout {
                      n141 = event-data() -> ()  [unwired: 1 in, 3 out]
                      n142 = local read "Manual Operation Control"() -> (w281:T3)
                      n143 = Unbundle By Name(w281) -> ("Linear.Step Length"=w285:dbl, "Rotative.Step Length"=w283:dbl)  [unwired: 1 out]
                      n144 = local read "System Status"() -> (w280:T4)
                      n145 = call <vilib>:"Read.vi"("Error In"=w290, "Xbox One Controller Ref"=w291) -> ("Error Out"=w289:errorcluster, "All Axis"=w286:T28, "Buttons"=w287:T18, "Xbox One Controller Ref"=w288:T9)  [unwired: 6 in]
                      n146 = Unbundle By Name(w286) -> ("Left Stick.X Axis"=w278:i32, "Left Stick.Y Axis"=w277:i32, "Right Stick.Y Axis"=w276:i32, "Triggers"=w275:i32)
                      n147 = Unbundle By Name(w287) -> ()  [unwired: 1 out]
                      n148 = Unbundle By Name(w280) -> ("Moving"=w279:bool)
                      n149 = Multiply(x=w283, y=1296000.0) -> (x*y=w272:dbl)
                      n150 = Bundle("X Axis"=w278, "Y Axis"=w277, "Y Axis"=w276, "Triggers"=w275) -> (w274:T30)  [unwired: 1 in]
                      n151 = Multiply(x=w285, y=1000.0) -> (x*y=w273:dbl)
                      n152 = case shown="True" w279 {
                        tunnel: w274 -> [_ w306]
                        tunnel: w273 -> [_ w308]
                        tunnel: w272 -> [_ w307]
                        frame False {
                        }
                        frame True {
                          # "start a relative movement"
                          n153 = Absolute Value(x=w306) -> (abs(x)=w311:T30)
                          n154 = Greater Than 0?(x=w306) -> (x > 0?=w304:T31)
                          n155 = Greater?(x=w311, y=5000) -> (0:w309:T31)
                          n156 = Cluster To Array(cluster=w309) -> (array=w301:bool[])
                          n157 = Cluster To Array(cluster=w304) -> (array=w300:bool[])
                          n158 = Array Size(array=w301) -> (size(s)=w305:i32)
                          n159 = for {
                            N: w305 -> [_]
                            tunnel: w301 -> [w321] mode=indexing
                            tunnel: w308 -> [w320]
                            tunnel: w307 -> [w319]
                            tunnel: [w318] -> w302 mode=indexing
                            n160 = Select(t=w319, s=w321, f=w320) -> (s? t:f=w318:dbl)
                          }
                          n161 = for {
                            N: w305 -> [_]
                            tunnel: w302 -> [w313] mode=indexing
                            tunnel: w300 -> [w314] mode=indexing
                            tunnel: [w312] -> w303 mode=indexing
                            n162 = case shown="False" w314 {
                              tunnel: w313 -> [w316 w317]
                              tunnel: [w315 w317] -> w312
                              frame False {
                                n163 = Negate(x=w316) -> (-x=w315:dbl)
                              }
                              frame True {
                              }
                            }
                          }
                          n164 = local read "Motor hModule"() -> (w299:i32)
                          n165 = Array To Cluster(array=w303) -> (cluster=w297:T32)
                          n166 = Unbundle By Name(w297) -> ("[0]"=w296:dbl, "[0]"=w295:dbl, "[0]"=w294:dbl, "[0]"=w293:dbl)
                          n167 = Bundle By Name(cluster=T7 {"PosX"=0, "PosY"=0, "PosZ"=0, "PosA"=0, "PosB"=0, "PosC"=0, "PosU"=0, "PosV"=0, "PosW"=0} ("RelPOS"), "PosX"=w296, "PosY"=w295, "PosZ"=w294, "PosA"=w293) -> (w292:T7)
                          n168 = call <userlib>:"mctl_MoveRel.vi"("RelPOS"=w292, "hModule In"=w299) -> ()  [unwired: 2 in, 2 out]
                        }
                      }
                    }
                    event User Event {
                      w323 = u32 3 items=["Restart", "Stop", "Break", "Abort"] ("Motion State")
                      n169 = event-data() -> ()  [unwired: 1 in, 5 out]
                      n170 = local read "Motor hModule"() -> (w322:i32)
                      n171 = call <userlib>:"mctl_SetMotionState.vi"("Motion State"=w323, "hModule In"=w322) -> ()  [unwired: 2 in, 2 out]
                    }
                    event User Event; "Exit Controller": Value Change {
                      n172 = event-data() -> ()  [unwired: 1 in, 3 out]
                      n173 = call <vilib>:"Read.vi"("Xbox One Controller Ref"=w330) -> ("Buttons"=w329:T18)  [unwired: 7 in, 3 out]
                      n174 = Unbundle By Name(w329) -> ("B"=w328:T20)
                      n175 = Or(x=w328, y="Exit Controller") -> (x .or. y?=w327:T20)
                    }
                  }
                }
              }
            }
            n176 = local read "Numeric 2"() -> (w249:dbl)
            n177 = Increment(x=w249) -> (x+1=→"Numeric 2":dbl)
          }
          event Mouse Up {
            w332 = u32 3 items=["Restart", "Stop", "Break", "Abort"] ("Motion State")
            # "Abort the movement the moment you lose the button.\nDon't use \"Break\" mode, which will cause step losses and other unexpected problem."
            n178 = event-data() -> ()  [unwired: 1 in, 8 out]
            n179 = local read "Motor hModule"() -> (w333:i32)
            n180 = call <userlib>:"mctl_SetMotionState.vi"("error in"=w335, "Motion State"=w332, "hModule In"=w333) -> ("error out"=w334:errorcluster)  [unwired: 1 in, 1 out]
          }
          event "Stop Motion": Mouse Up {
            # "Abort movement that is happening with no step losses"
            n181 = event-data() -> ()  [unwired: 1 in, 8 out]
            n182 = flat-sequence {
              tunnel: [w338] -> w336
              frame #0 {
                n183 = local write "Auto Run"(FALSE ("Auto Run")) -> ()
              }
              frame #1 {
                w339 = u32 3 items=["Restart", "Stop", "Break", "Abort"] ("Motion State")
                n184 = local read "Motor hModule"() -> (w340:i32)
                n185 = call <userlib>:"mctl_SetMotionState.vi"("Motion State"=w339, "hModule In"=w340) -> ("error out"=w338:errorcluster)  [unwired: 2 in, 1 out]
              }
            }
          }
          event "Reset Motion": Mouse Up {
            # "This function performs a reset of the machine control and the Motion Control DLL. The startup condition of the control is restored. A currently executed motion will be aborted immediately. Depending from the type of the connected control other, specific functions are executed. After calling the reset function, the machine resides in a \"Ready for operation\" state."
            n186 = event-data() -> ()  [unwired: 1 in, 8 out]
            n187 = local read "Motor hModule"() -> (w342:i32)
            n188 = call <userlib>:"mctl_Reset.vi"("hModule In"=w342) -> ("error out"=w341:errorcluster)  [unwired: 3 in, 1 out]
          }
          event "Reference": Mouse Up; User Event {
            n189 = event-data() -> ()  [unwired: 1 in, 3 out]
            n190 = call <vilib>:"Read.vi"("Error In"=w346, "Xbox One Controller Ref"=w347) -> ("Buttons"=w348:T18)  [unwired: 6 in, 3 out]
            n191 = Unbundle By Name(w348) -> ("Y"=w344:T22)
            n192 = Or(x="Reference", y=w344) -> (x .or. y?=w343:T22)
            n193 = case shown="True" w343 {
              tunnel: [errorcluster {"status"=FALSE, "code"=0, "source"=""} ("error out") w355] -> w349
              frame False {
              }
              frame True {
                # "The override is an additional velocity correction factor which is reckoned up with the current set velocities. \n\nThis function is used to set the override value of the Motion Control."
                # "Maybe move back to the zero point?"
                # "referrence run ?"
                # "set override"
                # "set vel"
                # "get vel"
                n194 = local read "Motor hModule"() -> (w360:i32)
                n195 = call <userlib>:"mctl_GetConfiguration.vi"("hModule In"=w360) -> ("error out"=w351:errorcluster, "Configuration"=w386:T33, "hModule Out"=w387:u32)  [unwired: 2 in]
                n196 = Unbundle By Name(w386) -> ("AxisConfig.AxisConfig 0.In Use"=w385:bool, "AxisConfig.AxisConfig 1.In Use"=w384:bool, "AxisConfig.AxisConfig 2.In Use"=w383:bool, "AxisConfig.AxisConfig 3.In Use"=w382:bool, "AxisConfig.AxisConfig 4.In Use"=w381:bool, "AxisConfig.AxisConfig 5.In Use"=w359:bool, "AxisConfig.AxisConfig 6.In Use"=w358:bool, "AxisConfig.AxisConfig 7.In Use"=w357:bool, "AxisConfig.AxisConfig 8.In Use"=w356:bool)
                n197 = local read "Manual Operation Control"() -> (w361:T3)
                n198 = Bundle("In Use"=w385, "In Use"=w384, "In Use"=w383, "In Use"=w382, "In Use"=w381, "In Use"=w359, "In Use"=w358, "In Use"=w357, "In Use"=w356) -> (w380:T34)  [unwired: 1 in]
                n199 = Unbundle By Name(w361) -> ("Speed Override (%)"=w366:dbl, "Linear.Speed"=w377:dbl, "Rotative.Speed"=w376:dbl)
                n200 = call <userlib>:"mctl_Reference.vi"("error in"=w351, "Reference Axis"=w380, "hModule In"=w387) -> ("error out"=w354:errorcluster, "hModule Out"=w365:u32)  [unwired: 1 in]
                n201 = Multiply(x=w377, y=1000.0) -> (x*y=w375:dbl)
                n202 = Multiply(x=w376, y=1296000.0) -> (x*y=w374:dbl)
                n203 = Multiply(x=75.0, y=1000.0) -> (x*y=w371:dbl)
                n204 = Multiply(x=2.8, y=1296000.0) -> (x*y=w370:dbl)
                n205 = call <userlib>:"mctl_GetVelocity.vi"("error in"=w354, "hModule In"=w365) -> ("error out"=w353:errorcluster, "Velocity"=w364:T16, "hModule Out"=w363:u32)  [unwired: 1 in]
                n206 = Bundle By Name(cluster=w364, "LiNormVel"=w375, "DrNormVel"=w374, "LiFastVel"=w371, "DrFastVel"=w370) -> (w367:T16)
                n207 = call <userlib>:"mctl_SetVelocity.vi"("error in"=w353, "Velocity"=w367, "hModule In"=w363) -> ("error out"=w352:errorcluster, "hModule Out"=w362:u32)  [unwired: 1 in]
                n208 = call <userlib>:"mctl_SetOverride.vi"("error in"=w352, "Override %"=w366, "hModule In"=w362) -> ("error out"=w355:errorcluster)  [unwired: 1 in, 1 out]
              }
            }
          }
          event "Leave HWLS": Mouse Up {
            # "leave Hardware Limit Switch \n\nAfter activating a hardware limit switch during a movement, the machine stops and the power supply of the machine is switched off for security reasons. If the hardware limit switch is still active after the machine has switched off, it is difficult to set the machine into an operative state."
            n209 = event-data() -> ()  [unwired: 1 in, 8 out]
            n210 = local read "Motor hModule"() -> (w395:i32)
            n211 = call <userlib>:"mctl_GetConfiguration.vi"("hModule In"=w395) -> ("error out"=w388:errorcluster, "Configuration"=w402:T33, "hModule Out"=w396:u32)  [unwired: 2 in]
            n212 = Unbundle By Name(w402) -> ("AxisConfig.AxisConfig 0.In Use"=w401:bool, "AxisConfig.AxisConfig 1.In Use"=w400:bool, "AxisConfig.AxisConfig 2.In Use"=w399:bool, "AxisConfig.AxisConfig 3.In Use"=w398:bool, "AxisConfig.AxisConfig 4.In Use"=w397:bool, "AxisConfig.AxisConfig 5.In Use"=w393:bool, "AxisConfig.AxisConfig 6.In Use"=w392:bool, "AxisConfig.AxisConfig 7.In Use"=w391:bool, "AxisConfig.AxisConfig 8.In Use"=w390:bool)
            n213 = Bundle("In Use"=w401, "In Use"=w400, "In Use"=w399, "In Use"=w398, "In Use"=w397, "In Use"=w393, "In Use"=w392, "In Use"=w391, "In Use"=w390) -> (w389:T34)  [unwired: 1 in]
            n214 = call <userlib>:"mctl_LeaveHWLS.vi"("error in"=w388, "Axis leave Limit"=w389, "hModule In"=w396) -> ("error out"=w394:errorcluster)  [unwired: 1 in, 1 out]
          }
          event "Test Mode": Mouse Up {
            # "Remarks \n\nNormally a Motion Control requires the execution of a reference run before it is fully operative. Since the reference run is not executed it is not possible to take access to the various movement functions of the Motion Control.\n \nIn some cases, e.g. during the start-up phase of working with a machine, it may be useful to access the movement functions without the previous execution of a reference run. The function mctl_SetTestMode() activates the so called \"Test mode\" which simulates a reference run if the complying function mctl_Reference() is called. //The current positions of each axis become the new machine zero point. //\n\nIn addition, the permanent checking of the hardware limit switches is switched off. The checking of hardware limit switches is used to set the Motion Control into an error state immediately after the activation of at least one hardware limit switch.// This feature enables you to move one or several axes into the mechanical stop for test purposes. //"
            n215 = event-data() -> ()  [unwired: 1 in, 8 out]
            n216 = local read "Motor hModule"() -> (w404:i32)
            n217 = call <userlib>:"mctl_GetStatus.vi"("hModule In"=w404) -> ("error out"=w405:errorcluster, "Status"=w409:T10, "hModule Out"=w406:u32)  [unwired: 2 in]
            n218 = Unbundle By Name(w409) -> ("Common.INTESTMODE"=w408:bool)
            n219 = Not(x=w408) -> (.not. x?=w407:bool)
            n220 = call <userlib>:"mctl_SetTestMode.vi"("error in"=w405, "Test Mode"=w407, "hModule In"=w406) -> ("error out"=w403:errorcluster)  [unwired: 1 in, 1 out]
          }
          event Mouse Down {
            n221 = event-data() -> ()  [unwired: 1 in, 8 out]
            n222 = flat-sequence {
              tunnel: ["Abs Position"] -> w413
              frame #0 {
                n223 = Wait (ms)(milliseconds to wait=u32 5) -> ()  [unwired: 1 out]
              }
              frame #1 {
              }
            }
            n224 = for {
              N: 1 -> [_]
              tunnel: w413 -> [w423]
              tunnel: [w436] -> w414
              tunnel: [w419] -> w410
              tunnel: w411 -> [w417]
              w430 = 1000
              n225 = Unbundle By Name(w423) -> ("OK Button"=w437:bool)
              n226 = Unbundle By Name(w423) -> ("Normal Move"=w420:bool, "Fast Move"=w422:bool, "Pos X"=w433:dbl, "Pos Y"=w432:dbl, "Pos Z"=w431:dbl, "Pos A"=w429:dbl)
              n227 = case shown="True" w437 {
                tunnel: w423 -> [w452 w458]
                tunnel: [w452 w453] -> w436
                frame False {
                }
                frame True {
                  n228 = local read "System Status"() -> (w459:T4)
                  n229 = Unbundle By Name(w459) -> ("Axis X.Position"=w457:dbl, "Axis Y.Position"=w456:dbl, "Axis Z.Position"=w455:dbl, "Axis A.Position"=w454:dbl)
                  n230 = Bundle By Name(cluster=w458, "Pos X"=w457, "Pos Y"=w456, "Pos Z"=w455, "Pos A"=w454) -> (w453:T2)
                }
              }
              n231 = local read "Motor hModule"() -> (w418:i32)
              n232 = Compound Arithmetic op=OR(w420, w422) -> (w421:bool)
              n233 = Multiply(x=w433, y=w430) -> (x*y=w427:dbl)
              n234 = Multiply(x=w432, y=w430) -> (x*y=w426:dbl)
              n235 = Multiply(x=w431, y=w430) -> (x*y=w425:dbl)
              n236 = Multiply(x=w429, y=1296000) -> (x*y=w424:dbl)
              n237 = Bundle By Name(cluster=T7 {"PosX"=0, "PosY"=0, "PosZ"=0, "PosA"=0, "PosB"=0, "PosC"=0, "PosU"=0, "PosV"=0, "PosW"=0} ("Abs"), "PosX"=w427, "PosY"=w426, "PosZ"=w425, "PosA"=w424) -> (w434:T7)
              n238 = case shown="True" w421 {
                tunnel: w434 -> [_ w443]
                tunnel: w420 -> [_ w442]
                tunnel: [w438 w441] -> w419
                tunnel: w418 -> [_ w440]
                tunnel: w417 -> [w438 w439]
                frame False {
                }
                frame True {
                  n239 = case shown="True" w442 {
                    tunnel: w443 -> [w447 w451]
                    tunnel: [w446 w450] -> w441
                    tunnel: w440 -> [w445 w449]
                    tunnel: w439 -> [w444 w448]
                    frame False {
                      n240 = call <userlib>:"mctl_FastAbs.vi"("error in"=w444, "FastAbs"=w447, "hModule In"=w445) -> ("error out"=w446:errorcluster)  [unwired: 1 in, 1 out]
                    }
                    frame True {
                      n241 = call <userlib>:"mctl_MoveAbs.vi"("error in"=w448, "Abs"=w451, "hModule In"=w449) -> ("error out"=w450:errorcluster)  [unwired: 1 in, 1 out]
                    }
                  }
                }
              }
            }
            n242 = local write "Abs Position"(w414) -> ()
          }
          event Mouse Down {
            n243 = event-data() -> ()  [unwired: 1 in, 8 out]
            n244 = flat-sequence {
              tunnel: ["Rel Position"] -> w463
              frame #0 {
                n245 = Wait (ms)(milliseconds to wait=u32 5) -> ()  [unwired: 1 out]
              }
              frame #1 {
              }
            }
            n246 = for {
              N: 1 -> [_]
              tunnel: w463 -> [w473]
              tunnel: [w486] -> w464
              tunnel: [w469] -> w460
              tunnel: w461 -> [w467]
              w480 = 1000
              n247 = Unbundle By Name(w473) -> ("OK Button"=w487:bool)
              n248 = Unbundle By Name(w473) -> ("Normal Move"=w470:bool, "Fast Move"=w472:bool, "Pos X"=w483:dbl, "Pos Y"=w482:dbl, "Pos Z"=w481:dbl, "Pos A"=w479:dbl)
              n249 = case shown="True" w487 {
                tunnel: w473 -> [w502 w508]
                tunnel: [w502 w503] -> w486
                frame False {
                }
                frame True {
                  n250 = local read "System Status"() -> (w509:T4)
                  n251 = Unbundle By Name(w509) -> ("Axis X.Position"=w507:dbl, "Axis Y.Position"=w506:dbl, "Axis Z.Position"=w505:dbl, "Axis A.Position"=w504:dbl)
                  n252 = Bundle By Name(cluster=w508, "Pos X"=w507, "Pos Y"=w506, "Pos Z"=w505, "Pos A"=w504) -> (w503:T2)
                }
              }
              n253 = local read "Motor hModule"() -> (w468:i32)
              n254 = Compound Arithmetic op=OR(w470, w472) -> (w471:bool)
              n255 = Multiply(x=w483, y=w480) -> (x*y=w477:dbl)
              n256 = Multiply(x=w482, y=w480) -> (x*y=w476:dbl)
              n257 = Multiply(x=w481, y=w480) -> (x*y=w475:dbl)
              n258 = Multiply(x=w479, y=1296000) -> (x*y=w474:dbl)
              n259 = Bundle By Name(cluster=T7 {"PosX"=0, "PosY"=0, "PosZ"=0, "PosA"=0, "PosB"=0, "PosC"=0, "PosU"=0, "PosV"=0, "PosW"=0} ("Abs"), "PosX"=w477, "PosY"=w476, "PosZ"=w475, "PosA"=w474) -> (w484:T7)
              n260 = case shown="True" w471 {
                tunnel: w484 -> [_ w493]
                tunnel: w470 -> [_ w492]
                tunnel: [w488 w491] -> w469
                tunnel: w468 -> [_ w490]
                tunnel: w467 -> [w488 w489]
                frame False {
                }
                frame True {
                  n261 = case shown="False" w492 {
                    tunnel: w493 -> [w497 w501]
                    tunnel: [w496 w500] -> w491
                    tunnel: w490 -> [w495 w499]
                    tunnel: w489 -> [w494 w498]
                    frame False {
                      n262 = call <userlib>:"mctl_FastRel.vi"("error in"=w494, "FastRel"=w497, "hModule In"=w495) -> ("error out"=w496:errorcluster)  [unwired: 1 in, 1 out]
                    }
                    frame True {
                      n263 = call <userlib>:"mctl_MoveRel.vi"("error in"=w498, "RelPOS"=w501, "hModule In"=w499) -> ("error out"=w500:errorcluster)  [unwired: 1 in, 1 out]
                    }
                  }
                }
              }
            }
            n264 = local write "Rel Position"(w464) -> ()
          }
          event Value Change {
            n265 = event-data() -> ()  [unwired: 1 in, 6 out]
            n266 = local read "Manual Operation Control"() -> (w512:T3)
            n267 = local read "Motor hModule"() -> (w510:i32)
            n268 = call <userlib>:"mctl_GetVelocity.vi"("hModule In"=w510) -> ("error out"=w517:errorcluster, "Velocity"=w516:T16, "hModule Out"=w518:u32)  [unwired: 2 in]
            n269 = Unbundle By Name(w512) -> ("Speed Override (%)"=w513:dbl, "Linear.Speed"=w523:dbl, "Rotative.Speed"=w522:dbl)
            n270 = Multiply(x=w523, y=1000.0) -> (x*y=w521:dbl)
            n271 = Multiply(x=w522, y=1296000.0) -> (x*y=w520:dbl)
            n272 = Bundle By Name(cluster=w516, "LiNormVel"=w521, "DrNormVel"=w520) -> (w519:T16)
            n273 = call <userlib>:"mctl_SetVelocity.vi"("error in"=w517, "Velocity"=w519, "hModule In"=w518) -> ("error out"=w514:errorcluster, "hModule Out"=w515:u32)  [unwired: 1 in]
            n274 = call <userlib>:"mctl_SetOverride.vi"("error in"=w514, "Override %"=w513, "hModule In"=w515) -> ("error out"=w511:errorcluster)  [unwired: 1 in, 1 out]
          }
        }
      }
      n275 = call <vilib>:"Close.vi"("Error In"=w58, "Xbox One Controller Ref"=w57) -> ("Error Out"=w56:errorcluster)  [unwired: 9 in]
      n276 = call <vilib>:"Simple Error Handler.vi"("error in (no error)"=w56) -> ()  [unwired: 4 in, 5 out]
    }
    frame #3 {
      w527 = FALSE ("Stop")
      # "Exit system"
      # "Restore value changes"
      # "Record current position information to position_zy.txt"
      # "Record current path information to path record.txt"
      n277 = local read "System Status"() -> (w532:T4)
      n278 = local read "Motor hModule"() -> (w533:i32)
      n279 = call <vilib>:"Application Directory.vi"() -> ("Application Directory"=w549:path)
      n280 = local read "MotionLibrary Path"() -> (w553:path)
      n281 = local read "MotionIni File In"() -> (w552:path)
      n282 = Unbundle By Name(w532) -> ("Initialized"=w531:bool)
      n283 = Bundle("MotionLibrary Path"=w553, "MotionIni File In"=w552) -> (w551:T8)  [unwired: 1 in]
      n284 = Build Path(base path=w549, name or relative path="path record.txt") -> (appended path=w558:path)
      n285 = Open/Create/Replace File(file path (use dialog)=w558, operation (0:open)=T5."replace or create") -> (refnum out=w557:refnum<file>, error out=w555:errorcluster)  [unwired: 4 in, 1 out]
      n286 = case shown="True" w531 {
        tunnel: w533 -> [_ w560]
        frame False {
        }
        frame True {
          n287 = call <userlib>:"mctl_Exit.vi"("hModule In"=w560) -> ()  [unwired: 3 in, 2 out]
        }
      }
      n288 = Write to Binary File(file (use dialog)=w557, data=w551, error in=w555, 5:FALSE ("prepend array or string size? (T)")) -> (refnum out=w556:refnum<file>, error out=w554:errorcluster)  [unwired: 2 in, 1 out]
      n289 = Close File(refnum=w556, error in=w554) -> ()  [unwired: 2 out]
      n290 = call <vilib>:"Application Directory.vi"() -> ("Application Directory"=w546:path)
      n291 = local read "Abs Position"() -> (w542:T2)
      n292 = local read "Rel Position"() -> (w543:T2)
      n293 = property on="Initialize" class="Bool (strict)"("BoolText.Text"="Initialize" ("Boolean Text.Text")) -> ()  [unwired: 2 in, 2 out]
      n294 = Bundle("Abs Position"=w542, "Rel Position"=w543) -> (w544:cluster{"Abs Position":T2, "Rel Position":T2})  [unwired: 1 in]
      n295 = Build Path(base path=w546, name or relative path="position_zy.txt") -> (appended path=w537:path)
      n296 = local write "Auto Run"(w527) -> ()
      n297 = local write "Exit"(w527) -> ()
      n298 = Open/Create/Replace File(file path (use dialog)=w537, operation (0:open)=T5."replace or create") -> (refnum out=w538:refnum<file>, error out=w540:errorcluster)  [unwired: 4 in, 1 out]
      n299 = Write to Binary File(file (use dialog)=w538, data=w544, error in=w540, 5:FALSE ("prepend array or string size? (T)")) -> (refnum out=w539:refnum<file>, error out=w541:errorcluster)  [unwired: 2 in, 1 out]
      n300 = Close File(refnum=w539, error in=w541) -> ()  [unwired: 2 out]
      n301 = local write "System Status"(T4 {"Axis X"={"Position"=0.0, "Limit NEG"=FALSE, "Limit  POS"=FALSE}, "Axis Y"={"Position"=0.0, "Limit NEG"=FALSE, "Limit  POS"=FALSE}, "Axis Z"={"Position"=0.0, "Limit NEG"=FALSE, "Limit  POS"=FALSE}, "Axis A"={"Position"=0.0, "Limit NEG"=FALSE, "Limit  POS"=FALSE}, "Initialized"=FALSE, " Moving"=FALSE, "Busy"=FALSE, "Need Ref."=FALSE, "Power Fail"=FALSE, "Test Mode"=FALSE, "Linear Speed"=0.0, "Rotativ Speed"=0.0, "Error Information"=""} ("System Status")) -> ()
      n302 = local read "Manual Operation Control"() -> (w530:T3)
      n303 = Bundle By Name(cluster=w530, "Axis-A Movement"=FALSE) -> (w528:T3)
      n304 = local write "Manual Operation Control"(w528) -> ()
      n305 = local write "Numeric 2"(0.0 ("Numeric")) -> ()
    }
  }
